vi "EnvelopeSignal.vi"(6 "sampling info":cluster{"Fs":dbl, "#s":dbl}={"Fs"=10240.0, "#s"=10240.0}, 9 "amplitude":dbl=1.0 format="%#_13g", 10 "Fault (order)":dbl, 11 "Running Speed (RPM)":dbl) -> (1 "Waveform Chart 5":waveform(dbl)(graph)={"t0"=timestamp(0 s since 1904-01-01), "dt"=9.765625e-05, "Y"=array[10240 elements]}, 2 "Waveform":waveform(dbl), 3 "Fault (Hz)":dbl=96.25, 4 "natural resonance":dbl=2887.5)   [LabVIEW 2017, in "CmsAcquisition.lvlib"]
uses:
  <vilib>/addons/InsightCM/Devices/Shared/Cms/CmsAcquisition/CmsAcquisition.lvlib
  <vilib>/measure/NI_MABase.lvlib
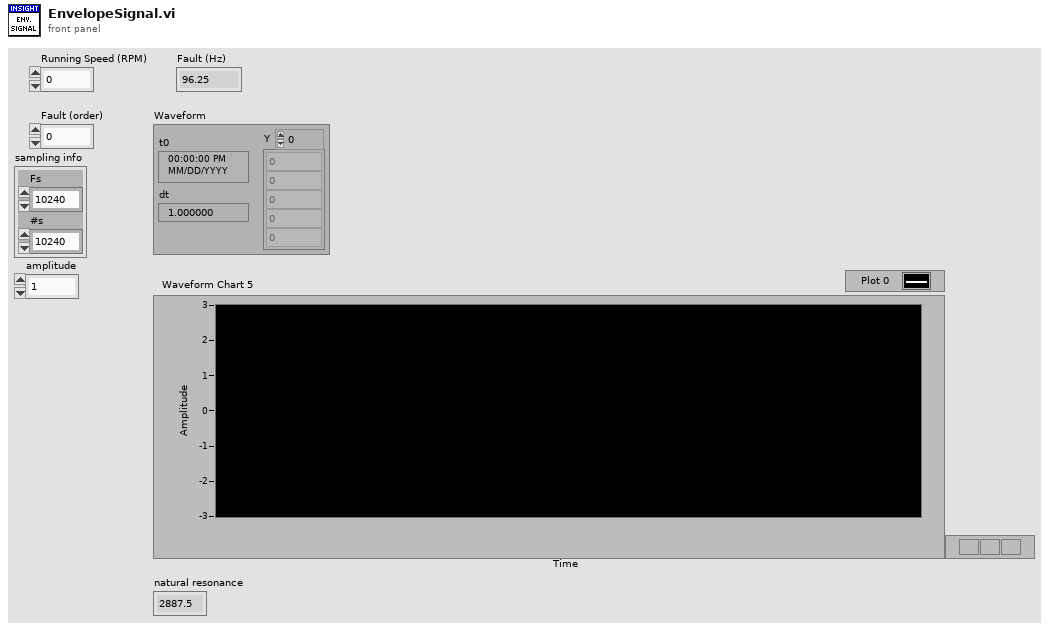
[diagram p1: front panel]
types:
  T1 = enum16{"Sine Wave", "Triangle Wave", "Square Wave", "Sawtooth Wave"}
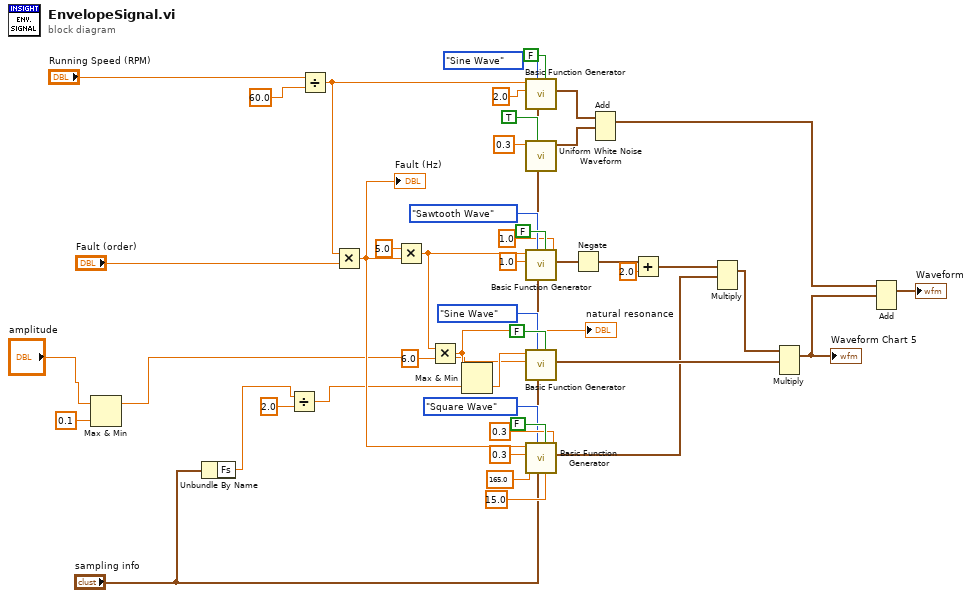
[diagram p0: block diagram]
diagram:
  n1 = Max & Min(x="amplitude", y=0.1) -> (max(x,y)=w1:dbl)  [unwired: 1 out]
  n2 = Unbundle By Name("sampling info") -> ("Fs"=w5:dbl)
  n3 = Divide(x=w5, y=2.0) -> (x/y=w4:dbl)
  n4 = Divide(x="Running Speed (RPM)", y=60.0) -> (x/y=w17:dbl)
  n5 = Multiply(x=w17, y="Fault (order)") -> (x*y=w41:dbl)
  "Fault (Hz)" <- w41
  n6 = Multiply(x=5.0 ("y"), y=w41) -> (x*y=w33:dbl)
  n7 = Multiply(x=w33, y=6.0) -> (x*y=w8:dbl)
  "natural resonance" <- w8
  n8 = Max & Min(x=w8, y=w4) -> (min(x,y)=w7:dbl)  [unwired: 1 out]
  n9 = call <vilib>:"Basic Function Generator.vi"("reset signal"=FALSE, "sampling info"="sampling info", "signal type"=T1."Sine Wave", "amplitude"=2.0, "frequency"=w17) -> ("signal out"=w14:waveform(dbl))  [unwired: 4 in, 2 out]
  n10 = call <vilib>:"Uniform White Noise Waveform.vi"("sampling info"="sampling info", "reset signal"=TRUE, "amplitude"=0.3) -> ("signal out"=w10:waveform(dbl))  [unwired: 7 in, 1 out]
  n11 = call <vilib>:"Basic Function Generator.vi"("offset"=1.0, "reset signal"=FALSE, "sampling info"="sampling info", "signal type"=T1."Sawtooth Wave", "amplitude"=1.0, "frequency"=w33) -> ("signal out"=w22:waveform(dbl))  [unwired: 3 in, 2 out]
  n12 = call <vilib>:"Basic Function Generator.vi"("reset signal"=FALSE, "sampling info"="sampling info", "signal type"=T1."Sine Wave", "amplitude"=w1, "frequency"=w7) -> ("signal out"=w36:waveform(dbl))  [unwired: 4 in, 2 out]
  n13 = call <vilib>:"Basic Function Generator.vi"("offset"=0.3, "square wave duty cycle (%)"=15.0 ("duty cycle (%)"), "reset signal"=FALSE, "sampling info"="sampling info", "signal type"=T1."Square Wave", "phase"=165.0, "amplitude"=0.3, "frequency"=w41) -> ("signal out"=w31:waveform(dbl))  [unwired: 1 in, 2 out]
  n14 = Negate(x=w22) -> (-x=w29:waveform(dbl))
  n15 = Add(1:w10, 2:w14) -> (0:w37:waveform(dbl))  [unwired: 1 in, 1 out]
  n16 = Add(x=w29, y=2.0) -> (x+y=w30:waveform(dbl))
  n17 = Multiply(1:w31, 2:w30) -> (0:w35:waveform(dbl))  [unwired: 1 in, 1 out]
  n18 = Multiply(1:w36, 2:w35) -> (0:w38:waveform(dbl))  [unwired: 1 in, 1 out]
  "Waveform Chart 5" <- w38
  n19 = Add(1:w38, 2:w37) -> (0:→"Waveform":waveform(dbl))  [unwired: 1 in, 1 out]
